vi "Sort Terminals.vi"(9 "Method Name":string, 10 "Flags":u32[](array[numeric]) format="%.0x", 11 "Ctrls[]":refnum<vi>[](array[refnum])) -> (0 "Error Out":refnum<class "SMOTerminal.lvclass">, 1 "Outputs":refnum<class "SMOTerminal.lvclass">[](array[class]), 2 "Inputs":refnum<class "SMOTerminal.lvclass">[](array[class]), 3 "Operand Out":refnum<class "SMOTerminal.lvclass">, 4 "Valid API":bool, 5 "Operand In":refnum<class "SMOTerminal.lvclass">)   [LabVIEW 2013, in "SMOTerminal.lvclass"]
uses:
  SMOTerminal.lvclass
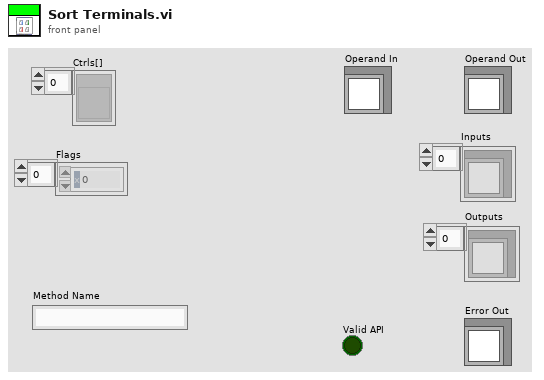
[diagram p1: front panel]
types:
  T1 = cluster{"Operand In":refnum<class "SMOTerminal.lvclass">, "Operand Out":refnum<class "SMOTerminal.lvclass">, "Error Out":refnum<class "SMOTerminal.lvclass">, "Inputs":refnum<class "SMOTerminal.lvclass">[], "Outputs":refnum<class "SMOTerminal.lvclass">[]}
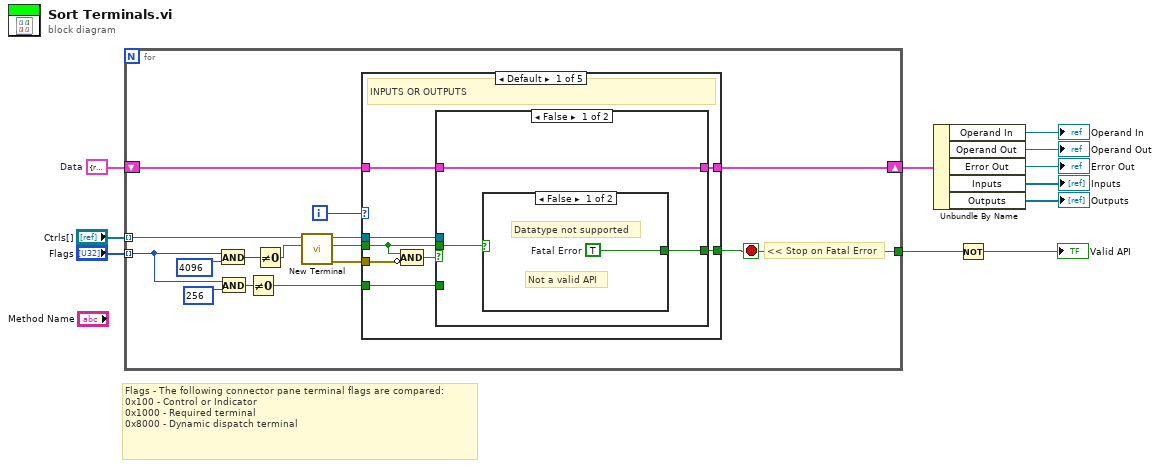
[diagram p0: block diagram]
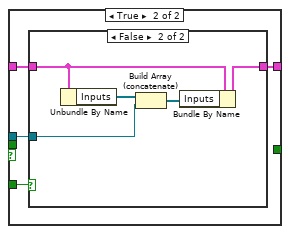
[diagram p3: hidden frame]
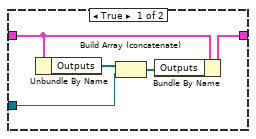
[diagram p4: hidden frame]
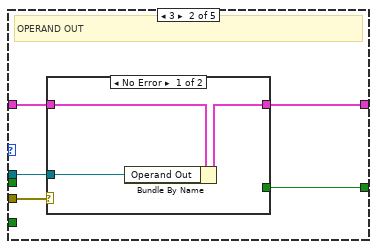
[diagram p5: hidden frame]
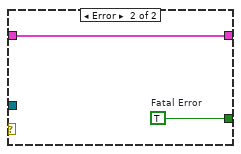
[diagram p6: hidden frame]
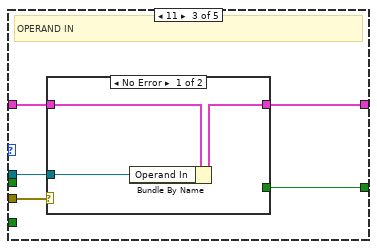
[diagram p7: hidden frame]
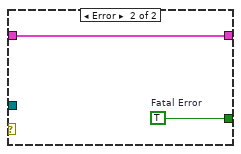
[diagram p8: hidden frame]
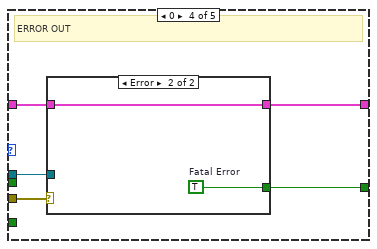
[diagram p9: hidden frame]
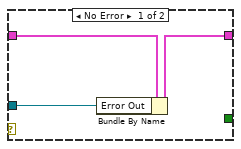
[diagram p10: hidden frame]
diagram:
  w9 = T1 {"Operand In"=refnum, "Operand Out"=refnum, "Error Out"=refnum, "Inputs"=[], "Outputs"=[]}  # Data
  # "Flags - The following connector pane terminal flags are compared:\n0x100 - Control or Indicator\n0x1000 - Required terminal\n0x8000 - Dynamic dispatch terminal"
  n1 = for {
    tunnel: "Ctrls[]" -> [w18] mode=indexing
    tunnel: "Flags" -> [w20] mode=indexing
    shift-right: [w22] -> w8
    shift-left: w9 -> [w23]
    tunnel: [w13] -> w2
    i -> [w24]
    stop <- w13 stop-if-true
    # "<< Stop on Fatal Error"
    n2 = And(x=w20, y=u32 4096) -> (x .and. y?=w25:u32)
    n3 = And(x=w20, y=u32 256) -> (x .and. y?=w19:u32)
    n4 = Not Equal To 0?(x=w19) -> (x != 0?=w12:bool)
    n5 = Not Equal To 0?(x=w25) -> (x != 0?=w17:bool)
    n6 = call "New Terminal.vi"("Required"=w17, "Control Reference"=w18) -> ("error out"=w14:errorcluster, "Supported type"=w15:bool, "Terminal out"=w16:refnum<class "SMOTerminal.lvclass">)  [unwired: 7 in]
    n7 = case shown="Default" w24 {
      tunnel: w23 -> [w32 w57 w67 w77 w83]
      tunnel: [w31 w56 w66 w76 w83] -> w22
      tunnel: w16 -> [w27 w55 w65 w75 _]
      tunnel: w15 -> [w30 _ _ _ _]
      tunnel: w14 -> [w34 w54 w64 w74 _]
      tunnel: [w29 w53 w63 w73 _] -> w13
      tunnel: w12 -> [w28 _ _ _ _]
      frame Default {
        # "INPUTS OR OUTPUTS"
        n8 = Compound Arithmetic op=AND(w30, invert w34) -> (w33:bool)
        n9 = case shown="False" w33 {
          tunnel: w32 -> [w37 w41]
          tunnel: [w37 w40] -> w31
          tunnel: w30 -> [w36 _]
          tunnel: [w35 _] -> w29
          tunnel: w28 -> [_ w42]
          tunnel: w27 -> [_ w39]
          frame False {
            n10 = case shown="False" w36 {
              tunnel: [w38 _] -> w35
              frame False {
                w38 = TRUE  # Fatal Error
                # "Not a valid API"
                # "Datatype not supported"
              }
              frame True {
                # "Terminal not connected"
              }
            }
          }
          frame True {
            n11 = case shown="False" w42 {
              tunnel: w41 -> [w46 w51]
              tunnel: [w47 w52] -> w40
              tunnel: w39 -> [w43 w48]
              frame True {
                n12 = Unbundle By Name(w46) -> ("Outputs"=w45:refnum<class "SMOTerminal.lvclass">[])
                n13 = Build Array (concatenate)(w45, w43) -> (w44:refnum<class "SMOTerminal.lvclass">[])
                n14 = Bundle By Name(cluster=w46, "Outputs"=w44) -> (w47:T1)
              }
              frame False {
                n15 = Unbundle By Name(w51) -> ("Inputs"=w50:refnum<class "SMOTerminal.lvclass">[])
                n16 = Build Array (concatenate)(w50, w48) -> (w49:refnum<class "SMOTerminal.lvclass">[])
                n17 = Bundle By Name(cluster=w51, "Inputs"=w49) -> (w52:T1)
              }
            }
          }
        }
      }
      frame 3 {
        # "OPERAND OUT"
        n18 = case shown="No Error" w54 {
          tunnel: w57 -> [w60 w62]
          tunnel: [w59 w62] -> w56
          tunnel: w55 -> [w58 _]
          tunnel: [_ w61] -> w53
          frame No Error {
            n19 = Bundle By Name(cluster=w60, "Operand Out"=w58) -> (w59:T1)
          }
          frame Error {
            w61 = TRUE  # Fatal Error
          }
        }
      }
      frame 11 {
        # "OPERAND IN"
        n20 = case shown="No Error" w64 {
          tunnel: w67 -> [w70 w72]
          tunnel: [w69 w72] -> w66
          tunnel: w65 -> [w68 _]
          tunnel: [_ w71] -> w63
          frame No Error {
            n21 = Bundle By Name(cluster=w70, "Operand In"=w68) -> (w69:T1)
          }
          frame Error {
            w71 = TRUE  # Fatal Error
          }
        }
      }
      frame 0 {
        # "ERROR OUT"
        n22 = case shown="Error" w74 {
          tunnel: w77 -> [w80 w82]
          tunnel: [w79 w82] -> w76
          tunnel: w75 -> [w78 _]
          tunnel: [_ w81] -> w73
          frame No Error {
            n23 = Bundle By Name(cluster=w80, "Error Out"=w78) -> (w79:T1)
          }
          frame Error {
            w81 = TRUE  # Fatal Error
          }
        }
      }
      frame 8 {
        # "ERROR IN"
      }
    }
  }
  n24 = Unbundle By Name(w8) -> ("Operand In"=→"Operand In":refnum<class "SMOTerminal.lvclass">, "Operand Out"=→"Operand Out":refnum<class "SMOTerminal.lvclass">, "Error Out"=→"Error Out":refnum<class "SMOTerminal.lvclass">, "Inputs"=→"Inputs":refnum<class "SMOTerminal.lvclass">[], "Outputs"=→"Outputs":refnum<class "SMOTerminal.lvclass">[])
  n25 = Not(x=w2) -> (.not. x?=→"Valid API":bool)
